vi "GDSArray_FindCommonElement.vi"(2 "I32Array":i32[](array[numeric])) -> (16 "MostCommonElement":i32, 17 "NrOfApperences":i32)   [LabVIEW 2012]
doc: "Finds the most common array element in a 1D array."
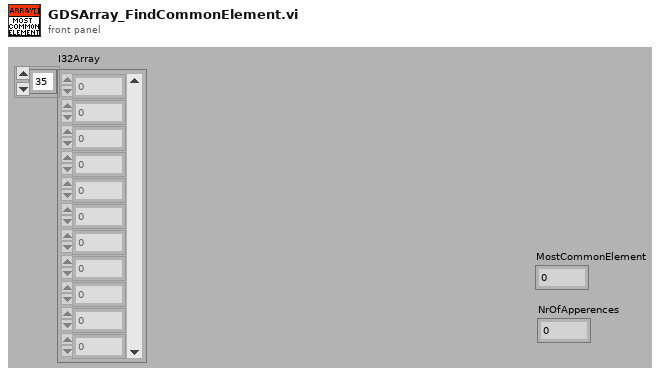
[diagram p1: front panel]
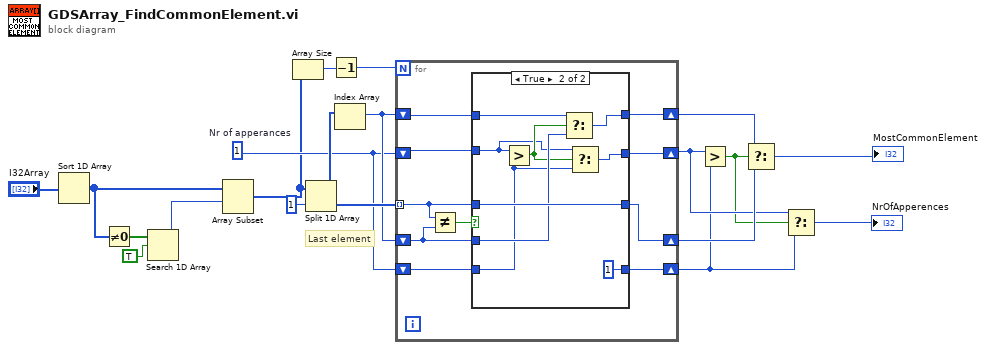
[diagram p0: block diagram]
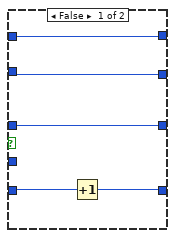
[diagram p2: hidden frame]
diagram:
  w11 = 1  # Nr of apperances
  # "Last element"
  n1 = Sort 1D Array(array="I32Array") -> (sorted array=w3:i32[])
  n2 = Not Equal To 0?(x=w3) -> (x != 0?=w5:bool[])
  n3 = Search 1D Array(1D array=w5, element=TRUE) -> (index of element=w1:i32)  [unwired: 1 in]
  n4 = Array Subset(array=w3, index=w1) -> (w2:i32[])  [unwired: 1 in]
  n5 = Array Size(array=w2) -> (size(s)=w16:i32)
  n6 = Split 1D Array(array=w2, index=1) -> (first subarray=w15:i32[], second subarray=w13:i32[])
  n7 = Decrement(x=w16) -> (x-1=w17:i32)
  n8 = Index Array(array=w15) -> (element=w12:i32)  [unwired: 1 in]
  n9 = for {
    N: w17 -> [_]
    shift-right: [w22] -> w10
    shift-left: w12 -> [w24]
    shift-right: [w21] -> w8
    shift-left: w11 -> [w25]
    tunnel: w13 -> [w29] mode=indexing
    shift-right: [w28] -> w9
    shift-left: w12 -> [w23]
    shift-right: [w27] -> w7
    shift-left: w11 -> [w26]
    n10 = Not Equal?(x=w29, y=w23) -> (x != y?=w30:bool)
    n11 = case shown="True" w30 {
      tunnel: w29 -> [w33 w44]
      tunnel: [w33 w44] -> w28
      tunnel: [w31 1 ("Nr of apperances")] -> w27
      tunnel: w26 -> [w32 w37]
      tunnel: w25 -> [w34 w38]
      tunnel: w24 -> [w35 w43]
      tunnel: w23 -> [_ w42]
      tunnel: [w35 w40] -> w22
      tunnel: [w34 w36] -> w21
      frame False {
        n12 = Increment(x=w32) -> (x+1=w31:i32)
      }
      frame True {
        n13 = Greater?(x=w38, y=w37) -> (0:w39:bool)
        n14 = Select(t=w43, s=w39, f=w42) -> (s? t:f=w40:i32)
        n15 = Select(t=w38, s=w39, f=w37) -> (s? t:f=w36:i32)
      }
    }
  }
  n16 = Greater?(x=w8, y=w7) -> (0:w6:bool)
  n17 = Select(t=w10, s=w6, f=w9) -> (s? t:f=→"MostCommonElement":i32)
  n18 = Select(t=w8, s=w6, f=w7) -> (s? t:f=→"NrOfApperences":i32)
